vi "MRFillLevelSafety.vi"(6 "fill level [l]":dbl, 7 "Valve":bool, 8 "enable":bool, 9 "Heating":bool, 10 "Circulation":bool, 11 "Pump":bool) -> (0 "max level":bool, 1 "Heating":bool, 2 "Circulation":bool, 3 "Pump":bool, 4 "min level":bool, 5 "Valve":bool)   [LabVIEW 2011]
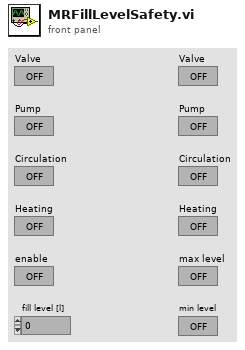
[diagram p1: front panel]
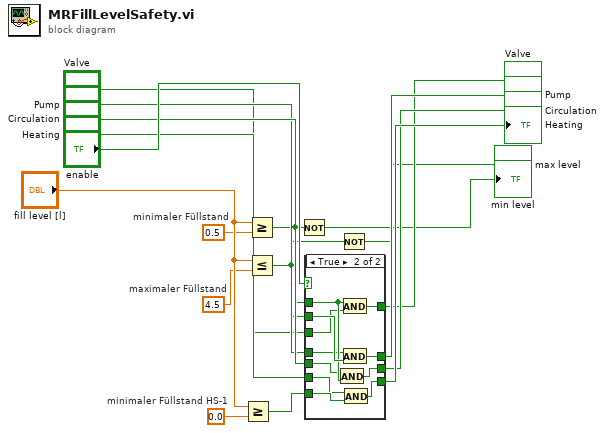
[diagram p0: block diagram]
diagram:
  w8 = 0.0  # minimaler Füllstand HS-1
  w2 = 0.5  # minimaler Füllstand
  w1 = 4.5  # maximaler Füllstand
  n1 = Greater Or Equal?(x="fill level [l]", y=w8) -> (x >= y?=w9:bool)
  n2 = Greater Or Equal?(x="fill level [l]", y=w2) -> (x >= y?=w5:bool)
  n3 = Less Or Equal?(x="fill level [l]", y=w1) -> (x <= y?=w3:bool)
  n4 = Not(x=w5) -> (.not. x?=→"min level":bool)
  n5 = case shown="True" "enable" {
    tunnel: w3 -> [_ w33]
    tunnel: w5 -> [_ w31]
    tunnel: w9 -> [_ w32]
    tunnel: "Valve" -> [w19 w30]
    tunnel: "Pump" -> [w20 w29]
    tunnel: "Circulation" -> [w21 w28]
    tunnel: "Heating" -> [w22 w27]
    tunnel: [w19 w26] -> w14
    tunnel: [w20 w25] -> w15
    tunnel: [w21 w24] -> w16
    tunnel: [w22 w23] -> w17
    frame False {
    }
    frame True {
      n6 = And(x=w28, y=w31) -> (x .and. y?=w24:bool)
      n7 = And(x=w31, y=w30) -> (x .and. y?=w26:bool)
      n8 = And(x=w29, y=w33) -> (x .and. y?=w25:bool)
      n9 = And(x=w27, y=w32) -> (x .and. y?=w23:bool)
    }
  }
  "Heating" <- w17
  "Circulation" <- w16
  "Pump" <- w15
  "Valve" <- w14
  n10 = Not(x=w3) -> (.not. x?=→"max level":bool)
